vi "MSGR VIServer Send.vi"(6 "Write?":bool, 9 "Parameters":string, 10 "Msg":string, 11 "MSGR Q name":T1) -> ()   [LabVIEW 2018]
doc: "MIT License\n\nCopyright (c) 2020 RichardLGP5\n\nPermission is hereby granted, free of charge, to any person obtaining a copy\nof this software and associated documentation files (the \"Software\"), to deal\nin the Software without restriction, including without limitation the rights\nto use, copy, modify, merge, publish, distribute, sublicense, and/or sell\ncopies of the Software, and to permit persons to whom the Software is\nfurnished to do so, subject to the following conditions:\n\nThe above copyright notice and this permission notice shall be included in all\ncopies or substantial portions of the Software.\n\nTHE SOFTWARE IS PROVIDED \"AS IS\", WITHOUT WARRANTY OF ANY KIND, EXPRESS OR\nIMPLIED, INCLUDING BUT NOT LIMITED TO THE WARRANTIES OF MERCHANTABILITY,\nFITNESS FOR A PARTICULAR PURPOSE AND NONINFRINGEMENT. IN NO EVENT SHALL THE\nAUTHORS OR COPYRIGHT HOLDERS BE LIABLE FOR ANY CLAIM, DAMAGES OR OTHER\nLIABILITY, WHETHER IN AN ACTION OF CONTRACT, TORT OR OTHERWISE, ARISING FROM,\nOUT OF OR IN CONNECTION WITH THE SOFTWARE OR THE USE OR OTHER DEALINGS IN THE\nSOFTWARE."
uses:
  MSGR Q Name TypeDef.ctl
  MSGR Get Q.vi
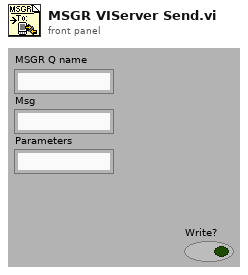
[diagram p1: front panel]
types:
  T1 = typedef "MSGR Q Name TypeDef.ctl" = string
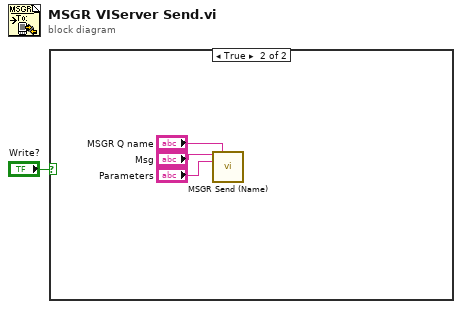
[diagram p0: block diagram]
diagram:
  n1 = case shown="True" "Write?" {
    frame False {
    }
    frame True {
      n2 = call "MSGR Send (Name).vi"("Msg"="Msg", "MSGR Q name"="MSGR Q name", "Parameters"="Parameters") -> ()  [unwired: 11 in, 2 out]
    }
  }
